vi "CR test.vi"() -> ()   [LabVIEW 2021]
uses:
  Data Model/ELAN Data Model/Type Definitions/Value full.ctl
  Data Unit/ELAN PC Data Unit/Elan units.ctl
  Data Unit/ELAN PC Data Unit/Elan measured variable.ctl
  Data Unit/ELAN PC Data Unit/Elan channel state.ctl
  enums/main_prog_state.ctl
  enums/init_state.ctl
  Master CR.lvclass
  Param/TCP Param/TCP Param.lvclass
  D:/my_projects/projects/Algorithms/Labview/21/Master CR/Param/Param.lvclass
  Master CR.lvclass/Master CR.ctl
  Param/Param.lvclass/Param.ctl
  Param/TCP Param/TCP Param.lvclass/TCP Param.ctl
  <vilib>/Platform/TimedLoop/XDataNode/timing_clust.ctl
  <vilib>/Platform/TimedLoop/XDataNode/nitl_modes.ctl
  <vilib>/Platform/TimedLoop/XDataNode/wakeup.ctl
  Data Model/ELAN Data Model/ELAN Data Model.lvclass
  enums/close_state.ctl
  <vilib>/Platform/TimedLoop/XDataNode/XDataNode.xnode
  Modbus_v121c/Data Model/Device Data Model.lvclass
  <vilib>/Platform/TimedLoop/XDataNode/XDNodeRunTimeDep.lvlib
  enums/Param_MB test.lvlib
  Param/Param.lvclass
  Data Unit/ELAN PC Data Unit/ELAN PDU.lvclass
panel:
  out "Values":T1[][](array[typedef]) {"Value"."Value" format="%#_6f"}
  in  "Write":bool
  in  "Read":bool
  out "connects":bool[](array[boolean])
  out "DI":bool[][](array[boolean])
  out "AI":u16[][](array[numeric])
  in  "DO":bool[][](array[boolean])
  in  "AOint":u16[][](array[numeric])
  out "comm error":errorcluster
  out "initialise error":errorcluster
  in  "EP_on":bool
  in  "tick":i64=100 caption="Время цикла основной программы" min=5 max=500 step=1
  in  "stop":bool
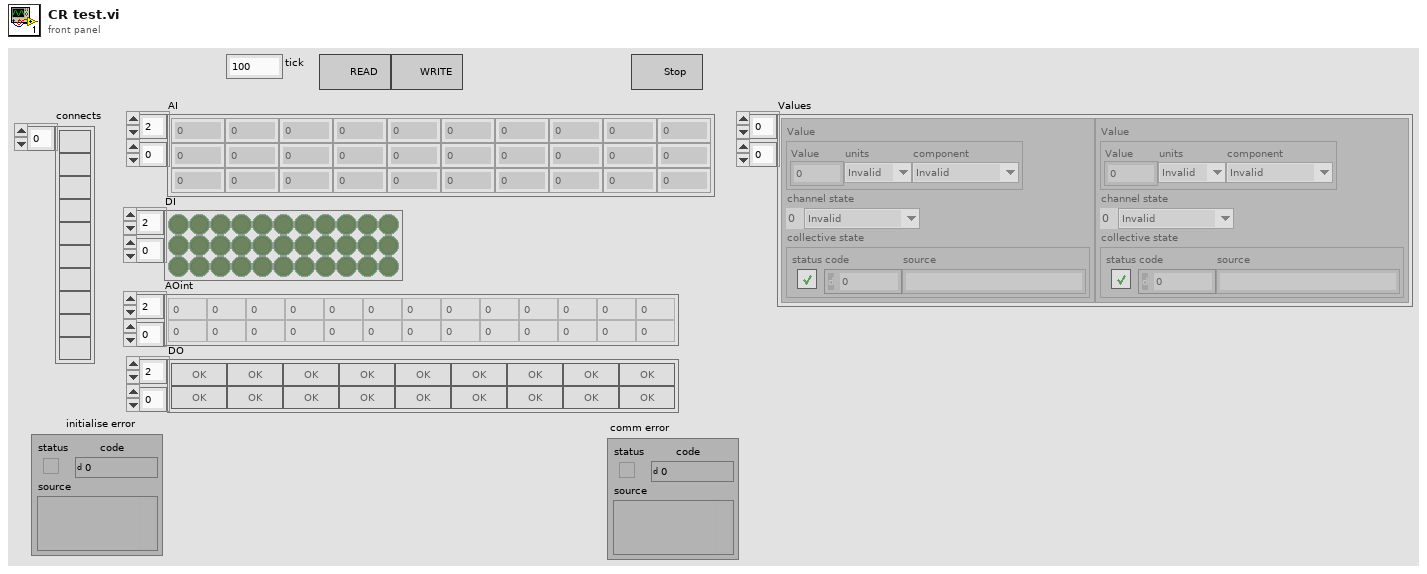
[diagram p1: front panel]
types:
  T1 = typedef "ELAN Data Model.lvclass/Value full.ctl" = cluster{"Value":cluster{"Value":sgl, "units":T2, "component":T3}, "channel state":T4, "collective state":errorcluster}
  T2 = typedef "ELAN PDU.lvclass/Elan units.ctl" = enum16{"Invalid", "no dimension", "ppm", "ppb", "vpm", "ppm C1", "ppm C3", "ppm C6", "mg C/m3", "mg/m3", "%", "% vol", "% of measuring range", "% saturation", "%/°C", "%/K", "% weight", "mV/pH", "mV/mbar", "nA/mbar", "S/m", "S/cm", "mS/m", "mS/cm", "мS/m", "мS/cm", "S", "min", "H", "Pa", "MA", "uV", "MV", "V", "mbar", "hPa", "Ml/min", "kOhm", "MOhm", "S1", "°C", "Hz", "pH", "ug/l", "mg/l", "l/min", "uA", "mg/dm3", "kPa", "kOhm*cm", "MOhm*cm", "°", "1/min", "1/m", "g/m3", "g/l", "% Vol C"}
  T3 = typedef "ELAN PDU.lvclass/Elan measured variable.ctl" = enum16{"Invalid", "no component", "CO", "CO2", "CH4 (Methan)", "C6H14 (Hexan)", "SO2", "NO", "NO2", "CHClF2 (R22)", "C3H8 (Propan)", "C4H10 (Butan)", "O2", "C5H12 (Pentan)", "CnHm (THC)", "P (process pressure)", "pH", "T (temperature)", "C2H4 (Ethen)", "C2H2 (Ethin)", "C3H6 (Propen)", "C4H6", "C4H8", "C2H6", "NH3 (Ammoniak)", "N2O", "C6H6 (Benzol)", "SF6", "CH3OH (Methanol)", "C2H5OH (Ethanol)", "CH2Cl2", "C2H4Cl2", "CH3Cl", "C2H4O", "H2O (water vapor)", "G/l (conductivity)", "C", "S", "N", "CF4", "COCl2 (phosgene)", "CHF3 (R23)", "C2F6 (R116)", "------ (self defined component)", "C2H3Cl", "H2 (Hydrogen)", "Ar", "He", "Cl2", "N2"}
  T4 = typedef "ELAN PDU.lvclass/Elan channel state.ctl" = enum16{"Invalid", "Warm-up", "Pause", "Standby", "Measure", "Zero calibration", "Adjust component slope", "Not yet defined1", "Adjust curve dip", "Adjust linearization sensitivity", "Adjust temperature compensation", "Adjust pressure compensation", "Adjust linearization zero", "Not yet defined2", "Autocal", "Adjust phase", "Zero calibration of O2 sensor", "Synchronous zero calibration", "Purging for synchronous zero calibration", "Adjust analog output", "Adjust analog input", "Autocal check"}
  T5 = cluster{"conn_timeout":i32, "reconn_timeout":i32, "N attempt max":i32, "t_reset_TTL":i32, "write_timeout":i32, "read_timeout":i32, "period":i32}[]
  T6 = cluster{"Remote IP Address":string, "Remote Port":u16}[]
  T7 = typedef "Param_MB test.lvlib/init_state.ctl" = enum16{"Init Data", "Init TMPs", "Init system DB", "Init data DB", "Read Enums", "Init arrays", "Init KFM", "Init Param", "Init AI param", "Init DI param", "Init AO param", "Init DO param", "Init ALR param", "Init save progs", "Read OPC param", "Init Shared Variables", "Init regulators", "Init heaters", "Init Y defs", "Exit"}
  T8 = typedef "Param_MB test.lvlib/main_prog_state.ctl" = enum16{"Read_AI_Param", "Read_DI_Param", "Read_AO_Param", "Read_DO_Param", "Read_ALR_ON_OFF", "Read_ALR_Param", "Read_Param", "Read_REG_Param", "Timers", "AI", "DI", "SendAItoScada", "SendDItoScada", "Alarms", "SendAItoDB", "SendDItoDB", "SendALRtoDB", "Messages", "Controls", "Control HT1", "QN_control", "QN", "QN_state", "Control EB3", "Outputs", "Exit"}
  T9 = cluster{"KFM":string[], "PAR":string[], "AI":string[], "DI":string[], "DI_fast":string[], "AO":string[], "Regs":string[], "DO":string[], "ALR":string[], "System":string[]}
  T10 = cluster{"Enums":cluster{"KFM":string[], "PAR":string[], "AI":string[], "DI":string[], "DI_fast":string[], "AO":string[], "Regs":string[], "DO":string[], "ALR":string[], "System":string[]}, "MBs":refnum<class "Master CR.lvclass">[]}
  T11 = cluster{"current time":timestamp, "Timer_1s":bool, "Timer_10s":bool, "Timer_1day":bool}
  T12 = typedef "XDNodeRunTimeDep.lvlib/timing_clust.ctl" = cluster{"Expected End [f-1]":u64, "Actual End [f-1]":u64, "Finished Late? [f-1]":bool, "Expected End [i-1]":u64, "Actual End [i-1]":u64, "Finished Late? [i-1]":bool, "Expected Start [i]":u64, "Actual Start [i]":u64, "Expected Start [f]":u64, "Actual Start [f]":u64, "Source Name":string, "Structure Name":string, "Period":i64, "Deadline":i64, "Offset":i64, "Start":i64, "Priority":i32, "Timeout":i32, "Mode":T13, "Wakeup Reason":T14, "Error":errorcluster, "Source Type":string, "Secondary Source Type":string, "Global End Time":u64, "Global Start Time":u64, "Frame Duration":u64, "Iteration Duration":u64, "Assigned CPU":i32, "I/O Scan Engine Mode":u32}
  T13 = typedef "XDNodeRunTimeDep.lvlib/nitl_modes.ctl" = enum32{"No Change", "Process missed periods, maintain original phase", "Discard missed periods, maintain original phase", "Process missed periods, ignore original phase", "Discard missed periods, ignore original phase"}
  T14 = typedef "XDNodeRunTimeDep.lvlib/wakeup.ctl" = enum32{"Normal", "Aborted", "Asynchronous wakeup", "Timing source error", "Timed loop error", "Timeout"}
  T15 = typedef "Param_MB test.lvlib/close_state.ctl" = enum16{"QN_state notifier", "QN_control_queue", "ALR notifires", "ALR", "DO notifires", "DO", "AO notifires", "AO", "DI notifres", "DI", "AI notifires", "AI", "OPC", "Param", "SaveMessageProg", "KFM DadaRef", "KFM Registers", "KFM StatusRef", "Exit"}
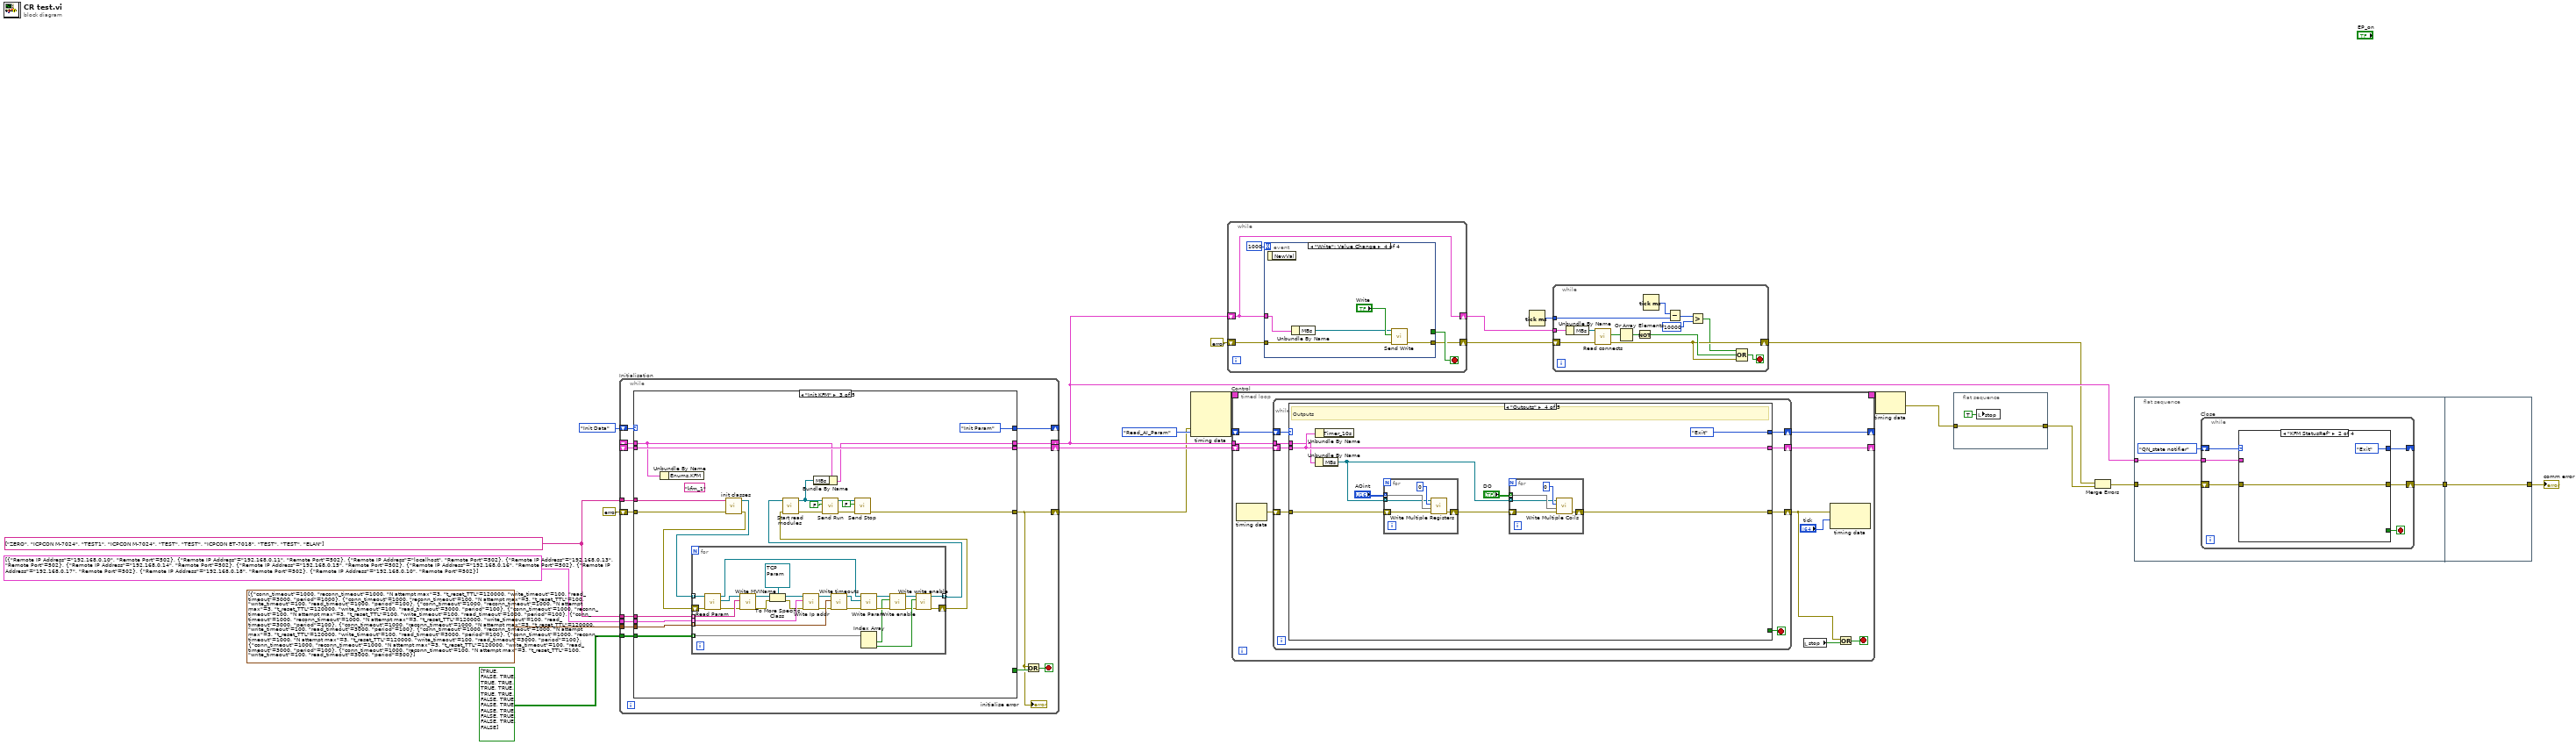
[diagram p0: block diagram]
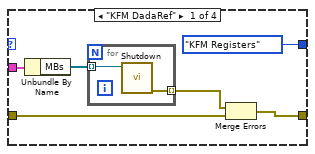
[diagram p2: hidden frame]
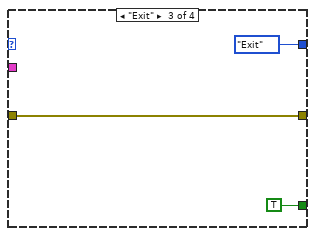
[diagram p3: hidden frame]
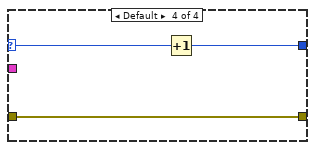
[diagram p4: hidden frame]
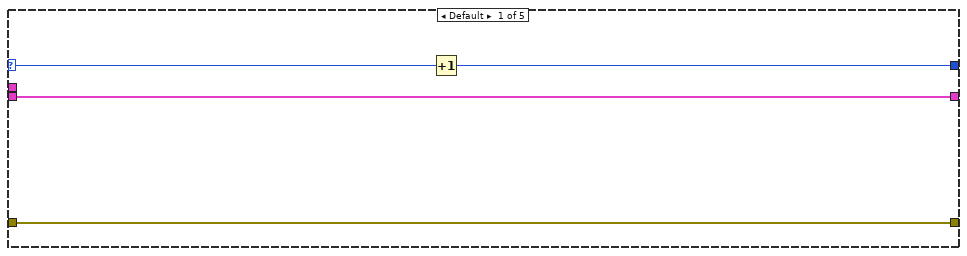
[diagram p5: hidden frame]
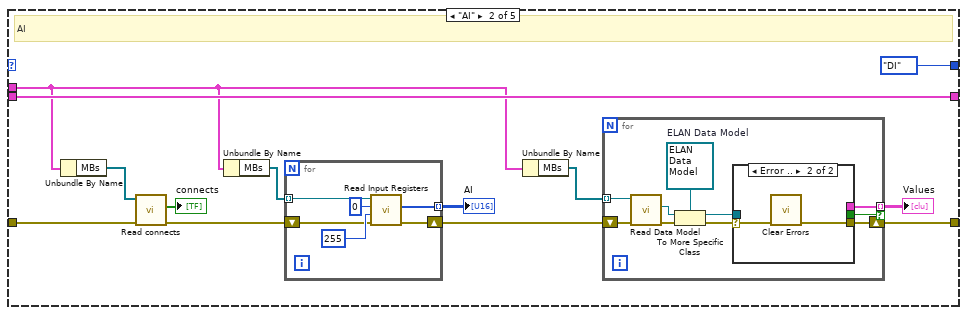
[diagram p6: hidden frame]
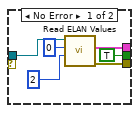
[diagram p7: hidden frame]
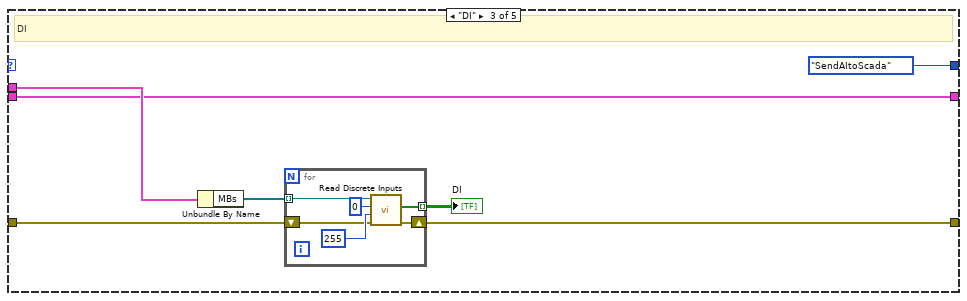
[diagram p8: hidden frame]
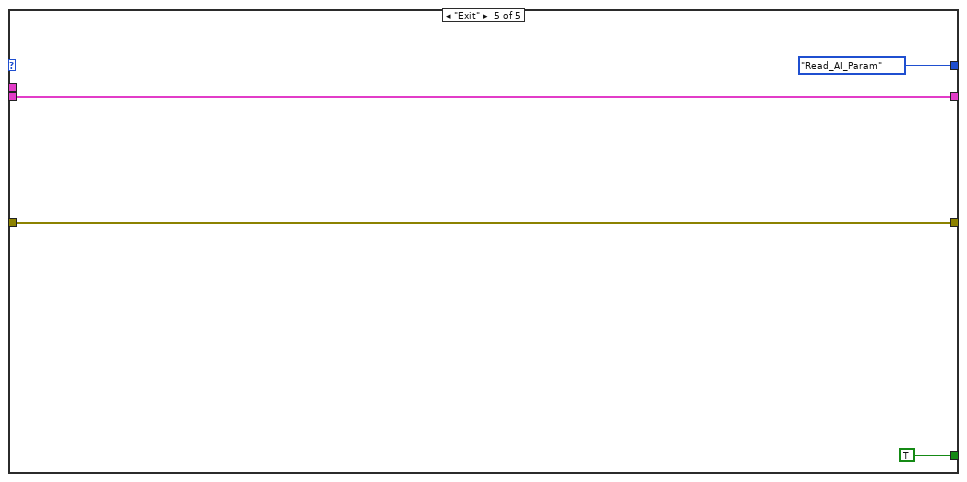
[diagram p9: hidden frame]
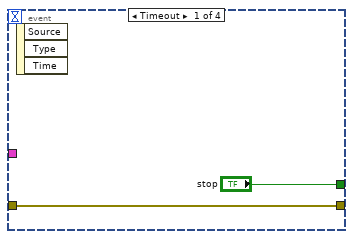
[diagram p10: hidden frame]
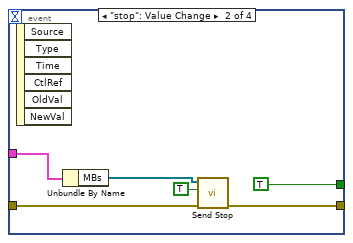
[diagram p11: hidden frame]
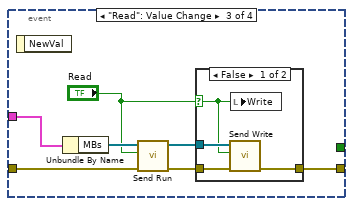
[diagram p12: hidden frame]
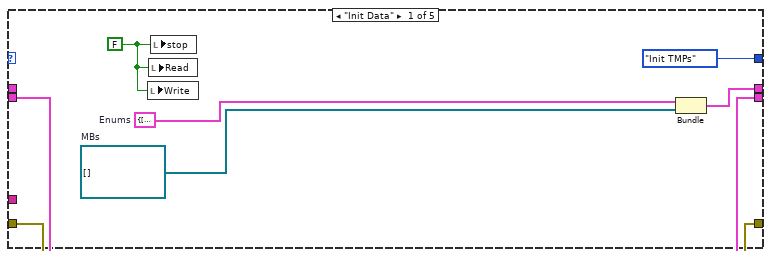
[diagram p14: hidden frame]
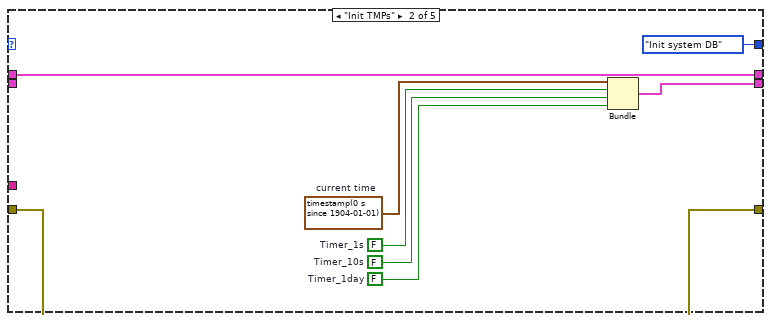
[diagram p15: hidden frame]
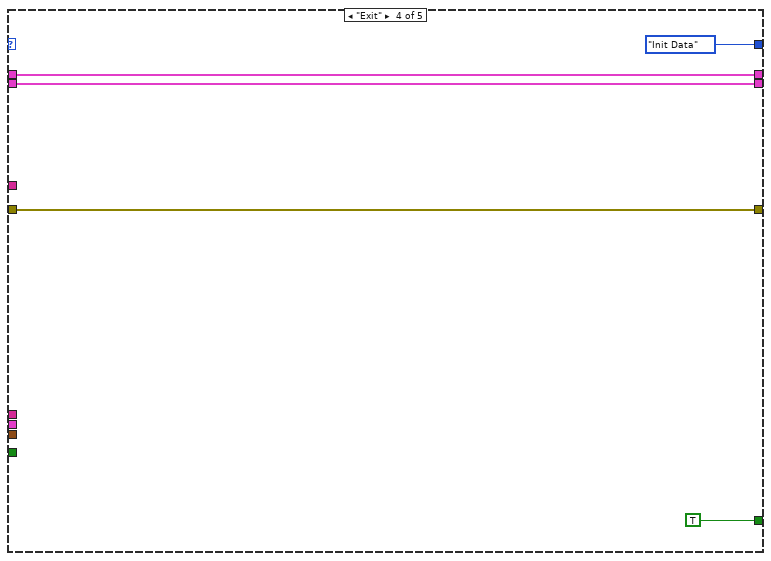
[diagram p16: hidden frame]
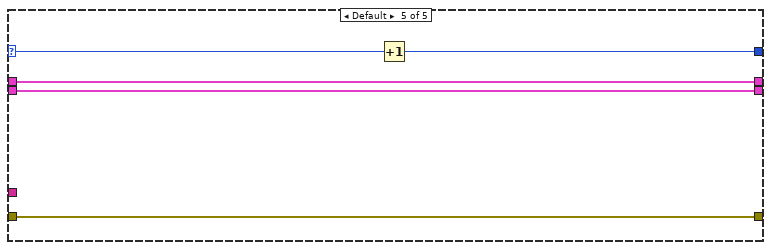
[diagram p17: hidden frame]
diagram:
  w8 = string[] ["ZERO", "ICPCON M-7024", "TEST1", "ICPCON M-7024", "TEST", "TEST", "ICPCON ET-7018", "TEST", "TEST", "ELAN"] ("MVIName")
  n1 = while "Initialisation" {
    shift-right: [w28] -> w7
    shift-left: errorcluster {"status"=FALSE, "code"=0, "source"=""} ("error out") -> [w34]
    shift-right: [w37] -> w13
    shift-left: _ -> [w35]
    shift-right: [w33] -> _
    shift-left: init_state."Init Data" -> [w36]
    shift-right: [w30] -> w16
    shift-left: _ -> [w29]
    tunnel: w8 -> [w27]
    tunnel: T6 [{"Remote IP Address"="192.168.0.10", "Remote Port"=502}, {"Remote IP Address"="192.168.0.11", "Remote Port"=502}, {"Remote IP Address"="localhost", "Remote Port"=502}, {"Remote IP Address"="192.168.0.13", "Remote Port"=502}, {"Remote IP Address"="192.168.0.14", "Remote Port"=502}, {"Remote IP Address"="192.168.0.15", "Remote Port"=502}, {"Remote IP Address"="192.168.0.16", "Remote Port"=502}, {"Remote IP Address"="192.168.0.17", "Remote Port"=502}, {"Remote IP Address"="192.168.0.18", "Remote Port"=502}, {"Remote IP Address"="192.168.0.10", "Remote Port"=502}] ("IP Address") -> [w26]
    tunnel: T5 [{"conn_timeout"=1000, "reconn_timeout"=1000, "N attempt max"=3, "t_reset_TTL"=120000, "write_timeout"=100, "read_timeout"=3000, "period"=1000}, {"conn_timeout"=1000, "reconn_timeout"=100, "N attempt max"=3, "t_reset_TTL"=100, "write_timeout"=100, "read_timeout"=1000, "period"=100}, {"conn_timeout"=1000, "reconn_timeout"=1000, "N attempt max"=3, "t_reset_TTL"=120000, "write_timeout"=100, "read_timeout"=3000, "period"=100}, {"conn_timeout"=1000, "reconn_timeout"=100, "N attempt max"=3, "t_reset_TTL"=100, "write_timeout"=100, "read_timeout"=1000, "period"=100}, {"conn_timeout"=1000, "reconn_timeout"=1000, "N attempt max"=3, "t_reset_TTL"=120000, "write_timeout"=100, "read_timeout"=3000, "period"=100}, {"conn_timeout"=1000, "reconn_timeout"=1000, "N attempt max"=3, "t_reset_TTL"=120000, "write_timeout"=100, "read_timeout"=3000, "period"=100}, {"conn_timeout"=1000, "reconn_timeout"=1000, "N attempt max"=3, "t_reset_TTL"=120000, "write_timeout"=100, "read_timeout"=3000, "period"=100}, {"conn_timeout"=1000, "reconn_timeout"=1000, "N attempt max"=3, "t_reset_TTL"=120000, "write_timeout"=100, "read_timeout"=3000, "period"=100}, {"conn_timeout"=1000, "reconn_timeout"=1000, "N attempt max"=3, "t_reset_TTL"=120000, "write_timeout"=100, "read_timeout"=3000, "period"=100}, {"conn_timeout"=1000, "reconn_timeout"=100, "N attempt max"=3, "t_reset_TTL"=100, "write_timeout"=100, "read_timeout"=3000, "period"=500}] ("timeouts") -> [w25]
    tunnel: bool[][] [[TRUE, FALSE], [TRUE, TRUE], [TRUE, TRUE], [TRUE, TRUE], [TRUE, FALSE], [TRUE, FALSE], [TRUE, FALSE], [TRUE, FALSE], [TRUE, FALSE], [TRUE, FALSE]] ("enable") -> [w24]
    tunnel: w8 -> [w23]
    stop <- w31 stop-if-true
    # "Initialisation"
    n2 = case shown="\"Init KFM\"" w36 {
      tunnel: [w42 w51 w53 w102 w105] -> w28
      selector: w36 -> [_ _ _ _ w108]
      tunnel: [w43 w50 w54 w103 w106] -> w37
      tunnel: w35 -> [_ w50 w71 w103 w106]
      tunnel: w34 -> [w42 w51 w70 w102 w105]
      tunnel: [init_state."Init TMPs" init_state."Init system DB" init_state."Init Param" init_state."Init Data" w107] -> w33
      tunnel: [_ _ _ TRUE _] -> w32
      tunnel: [w40 w49 w72 w100 w109] -> w30
      tunnel: w29 -> [w40 _ w72 w100 w109]
      tunnel: w27 -> [_ _ w65 _ _]
      tunnel: w26 -> [_ _ w64 _ _]
      tunnel: w25 -> [_ _ w63 _ _]
      tunnel: w24 -> [_ _ w62 _ _]
      tunnel: w23 -> [_ _ w61 _ _]
      frame "Init Data" {
        w38 = FALSE ("stop")
        w39 = refnum<class "Master CR.lvclass">[] []  # MBs
        w41 = T9 {"KFM"=[], "PAR"=[], "AI"=[], "DI"=[], "DI_fast"=[], "AO"=[], "Regs"=[], "DO"=[], "ALR"=[], "System"=[]}  # Enums
        n3 = local write "Write"(w38) -> ()
        n4 = local write "Read"(w38) -> ()
        n5 = local write "stop"(w38) -> ()
        n6 = Bundle("Enums"=w41, "MBs"=w39) -> (w43:T10)  [unwired: 1 in]
      }
      frame "Init TMPs" {
        w45 = FALSE  # Timer_10s
        w46 = FALSE  # Timer_1day
        w47 = FALSE  # Timer_1s
        w48 = timestamp(0 s since 1904-01-01)  # current time
        n7 = Bundle("current time"=w48, "Timer_1s"=w47, "Timer_10s"=w45, "Timer_1day"=w46) -> (w49:T11)  [unwired: 1 in]
      }
      frame "Init KFM" {
        (unwired) "kfm_1" ("KFMTable")
        n8 = Unbundle By Name(w71) -> ()  [unwired: 1 out]
        n9 = call "init classes.vi"("error in (no error)"=w70, "MVINames"=w61) -> ("error out"=w67:errorcluster, "MBs"=w69:refnum<class "Master CR.lvclass">[])  [unwired: 8 in]
        n10 = for {
          tunnel: w69 -> [w75] mode=indexing
          tunnel: w64 -> [w82] mode=indexing
          tunnel: w63 -> [w79] mode=indexing
          tunnel: w65 -> [w97] mode=indexing
          tunnel: w62 -> [w91] mode=indexing
          tunnel: [w87] -> w68 mode=indexing
          shift-right: [w86] -> w66
          shift-left: w67 -> [w99]
          n11 = call "Read Param.vi"("error in (no error)"=w99, "MB_TCP in"=w75) -> ("error out"=w95:errorcluster, "Param"=w74:refnum<class "Param.lvclass">, "MB_TCP out"=w94:refnum<class "Master CR.lvclass">)  [unwired: 7 in]
          n12 = call "Write MVIName.vi"("error in (no error)"=w95, "MVIName"=w97, "MB Param in"=w74) -> ("error out"=w84:errorcluster, "MB Param out"=w96:refnum<class "Param.lvclass">)  [unwired: 7 in]
          n13 = To More Specific Class(target class=refnum<class "TCP Param.lvclass"> refnum ("Param.lvlib:TCP Param.lvclass"), reference=w96, error in=w84) -> (specific class reference=w83:refnum<class "TCP Param.lvclass">, error out=w81:errorcluster)
          n14 = call "Write Ip addr.vi"("error in (no error)"=w81, "IP address"=w82, "MB Param in"=w83) -> ("error out"=w78:errorcluster, "MB Param out"=w80:refnum<class "TCP Param.lvclass">)  [unwired: 7 in]
          n15 = call "Write timeouts.vi"("error in (no error)"=w78, "timeouts"=w79, "MB Param in"=w80) -> ("error out"=w77:errorcluster, "MB Param out"=w76:refnum<class "TCP Param.lvclass">)  [unwired: 7 in]
          n16 = call "Write Param.vi"("error in (no error)"=w77, "Param"=w76, "MB_TCP in"=w94) -> ("error out"=w92:errorcluster, "MB_TCP out"=w93:refnum<class "Master CR.lvclass">)  [unwired: 7 in]
          n17 = Index Array(array=w91) -> (element #1=w90:bool, element #2=w89:bool)  [unwired: 2 in]
          n18 = call "Write enable.vi"("error in (no error)"=w92, "enable"=w90, "Master CR in"=w93) -> ("error out"=w88:errorcluster, "Master CR out"=w98:refnum<class "Master CR.lvclass">)  [unwired: 7 in]
          n19 = call "Write write enable.vi"("error in (no error)"=w88, "write enable"=w89, "Master CR in"=w98) -> ("error out"=w86:errorcluster, "Master CR out"=w87:refnum<class "Master CR.lvclass">)  [unwired: 7 in]
        }
        n20 = call "Start read modules.vi"("error in"=w66, "classes"=w68) -> ("error out"=w56:errorcluster, "classes initialised"=w55:refnum<class "Master CR.lvclass">[])  [unwired: 8 in]
        n21 = Bundle By Name(cluster=w71, "MBs"=w55) -> (w54:T10)
        n22 = call "Send Run.vi"("error in"=w56, "Run"=FALSE, "MCRs"=w55) -> ("error out"=w59:errorcluster, "MCRs out"=w60:refnum<class "Master CR.lvclass">[])  [unwired: 7 in]
        n23 = call "Send Stop.vi"("error in"=w59, "Stop"=FALSE ("Write"), "MCRs"=w60) -> ("error out"=w53:errorcluster)  [unwired: 7 in, 1 out]
      }
      frame "Exit" {
      }
      frame Default {
        n24 = Increment(x=w108) -> (x+1=w107:T7)
      }
    }
    "initialise error" <- w28
    n25 = Or(x=w28, y=w32) -> (x .or. y?=w31:bool)
  }
  n26 = node-c288(w7) -> (w22:T12)  [unwired: 3 in]
  n27 = while {
    shift-right: [w112] -> w4
    shift-left: errorcluster {"status"=FALSE, "code"=0, "source"=""} ("error out") -> [w111]
    shift-right: [w110] -> w3
    shift-left: w13 -> [w110]
    stop <- w113 stop-if-true
    n28 = event shown="[3] \"Write\": Value Change" {
      selector: _ -> [_ _ _ _]
      dyn-events: _ -> [_ _ _ _]
      timeout: 1000 -> [_ _ _ _]
      tunnel: ["stop" TRUE ("stop") _ _] -> w113
      tunnel: w110 -> [_ w117 w129 w139]
      tunnel: w111 -> [w115 w121 w128 w138]
      tunnel: [w115 w120 w123 w137] -> w112
      event Timeout {
        n29 = event-data() -> ()  [unwired: 1 in, 3 out]
      }
      event "stop": Value Change {
        n30 = event-data() -> ()  [unwired: 1 in, 6 out]
        n31 = Unbundle By Name(w117) -> ("MBs"=w118:refnum<class "Master CR.lvclass">[])
        n32 = call "Send Stop.vi"("error in"=w121, "Stop"=TRUE, "MCRs"=w118) -> ("error out"=w120:errorcluster)  [unwired: 7 in, 1 out]
      }
      event "Read": Value Change {
        n33 = event-data() -> ()  [unwired: 1 in, 1 out]
        n34 = Unbundle By Name(w129) -> ("MBs"=w127:refnum<class "Master CR.lvclass">[])
        n35 = call "Send Run.vi"("error in"=w128, "Run"="Read", "MCRs"=w127) -> ("error out"=w125:errorcluster, "MCRs out"=w124:refnum<class "Master CR.lvclass">[])  [unwired: 7 in]
        n36 = case shown="False" "Read" {
          selector: "Read" -> [w131 _]
          tunnel: w125 -> [w133 w134]
          tunnel: w124 -> [w132 _]
          tunnel: [w130 w134] -> w123
          frame False {
            n37 = call "Send Write.vi"("error in"=w133, "Write"=w131, "MCRs"=w132) -> ("error out"=w130:errorcluster)  [unwired: 7 in, 1 out]
            n38 = local write "Write"(w131) -> ()
          }
          frame True {
          }
        }
      }
      event "Write": Value Change {
        n39 = event-data() -> ()  [unwired: 1 in, 1 out]
        n40 = Unbundle By Name(w139) -> ("MBs"=w135:refnum<class "Master CR.lvclass">[])
        n41 = call "Send Write.vi"("error in"=w138, "Write"="Write", "MCRs"=w135) -> ("error out"=w137:errorcluster)  [unwired: 7 in, 1 out]
      }
    }
  }
  n42 = timed-loop "Control" {
    tunnel: w13 -> [w149]
    shift-right: [w147] -> _
    shift-left: w16 -> [w148]
    timing: w22 -> [_]
    timing-out: [_] -> w21
    shift-right: [w145] -> _
    shift-left: main_prog_state."Read_AI_Param" -> [w144]
    stop <- w142 stop-if-true
    n43 = node-c288() -> (w146:errorcluster)  [unwired: 1 in]
    n44 = while {
      tunnel: w149 -> [w157]
      shift-right: [w155] -> w147
      shift-left: w148 -> [w156]
      shift-right: [w150] -> w140
      shift-left: w146 -> [w154]
      shift-right: [w153] -> w145
      shift-left: w144 -> [w152]
      stop <- w151 stop-if-true
      n45 = case shown="\"Outputs\"" w152 {
        tunnel: w154 -> [w158 w173 w201 w217 w231]
        tunnel: w157 -> [_ w163 w204 w218 _]
        tunnel: w156 -> [w160 w171 w203 w219 w232]
        tunnel: [w160 w171 w203 w219 w232] -> w155
        selector: w152 -> [w161 _ _ _ _]
        tunnel: [w159 main_prog_state."DI" main_prog_state."SendAItoScada" main_prog_state."Exit" main_prog_state."Read_AI_Param"] -> w153
        tunnel: [_ _ _ _ TRUE] -> w151
        tunnel: [w158 w169 w200 w213 w231] -> w150
        frame Default {
          n46 = Increment(x=w161) -> (x+1=w159:T8)
        }
        frame "AI" {
          # "AI"
          n47 = Unbundle By Name(w163) -> ("MBs"=w172:refnum<class "Master CR.lvclass">[])
          n48 = call "Read connects.vi"("error in (no error)"=w173, "MCRs in"=w172) -> ("error out"=w166:errorcluster, "connects"=→"connects":bool[])  [unwired: 7 in, 1 out]
          n49 = Unbundle By Name(w163) -> ("MBs"=w164:refnum<class "Master CR.lvclass">[])
          n50 = for {
            tunnel: w164 -> [w176] mode=indexing
            shift-right: [w180] -> w165
            shift-left: w166 -> [w175]
            tunnel: [w177] -> w162 mode=indexing
            n51 = call "Read Input Registers.vi"("error in"=w175, "number of inputs"=u16 255 ("number of coils"), "starting address"=u16 0, "Master CR in"=w176) -> ("error out"=w180:errorcluster, "register values"=w177:u16[])  [unwired: 5 in, 1 out]
          }
          "AI" <- w162
          n52 = Unbundle By Name(w163) -> ("MBs"=w170:refnum<class "Master CR.lvclass">[])
          n53 = for {
            tunnel: w170 -> [w187] mode=indexing
            shift-right: [w190] -> w169
            shift-left: w165 -> [w188]
            tunnel: [w189] -> w167 mode=indexing if=w181
            w185 = refnum<class "ELAN Data Model.lvclass"> refnum  # ELAN Data Model
            n54 = call "Read Data Model.vi"("error in (no error)"=w188, "Master CR in"=w187) -> ("error out"=w186:errorcluster, "Data Model"=w184:refnum<class "Device Data Model.lvclass">)  [unwired: 7 in, 1 out]
            n55 = To More Specific Class(target class=w185, reference=w184, error in=w186) -> (specific class reference=w183:refnum<class "ELAN Data Model.lvclass">, error out=w182:errorcluster)
            n56 = case shown="Error .." w182 {
              selector: w182 -> [_ w198]
              tunnel: [w196 w197] -> w190
              tunnel: [w193 _] -> w189
              tunnel: w183 -> [w192 _]
              tunnel: [TRUE _] -> w181
              frame No Error {
                n57 = call-dynamic "Read ELAN Values.vi"("number of registers"=u16 2 ("number of coils"), "starting address"=u16 0, "standard data model in"=w192) -> ("error out"=w196:errorcluster, "Values"=w193:T1[])  [unwired: 6 in, 1 out]
              }
              frame Error {
                n58 = call <vilib>:"Clear Errors.vi"("error in (no error)"=w198) -> ("error out"=w197:errorcluster)  [unwired: 5 in, 1 out]
              }
            }
          }
          "Values" <- w167
        }
        frame "DI" {
          # "DI"
          n59 = Unbundle By Name(w204) -> ("MBs"=w202:refnum<class "Master CR.lvclass">[])
          n60 = for {
            tunnel: w202 -> [w207] mode=indexing
            shift-right: [w211] -> w200
            shift-left: w201 -> [w206]
            tunnel: [w208] -> w199 mode=indexing
            n61 = call "Read Discrete Inputs.vi"("error in"=w206, "number of inputs"=u16 255 ("number of coils"), "starting address"=u16 0, "Master CR in"=w207) -> ("error out"=w211:errorcluster, "discrete inputs"=w208:bool[])  [unwired: 5 in, 1 out]
          }
          "DI" <- w199
        }
        frame "Outputs" {
          # "Outputs"
          n62 = Unbundle By Name(w218) -> ("MBs"=w212:refnum<class "Master CR.lvclass">[])
          n63 = Unbundle By Name(w219) -> ()  [unwired: 1 out]
          n64 = for {
            tunnel: w212 -> [w226] mode=indexing
            shift-right: [w230] -> w214
            shift-left: w217 -> [w227]
            tunnel: "AOint" -> [w228] mode=indexing
            n65 = call-dynamic "Write Multiple Registers.vi"("error in"=w227, "register values"=w228, "starting address"=u16 0, "Master CR in"=w226) -> ("error out"=w230:errorcluster)  [unwired: 6 in, 1 out]
          }
          n66 = for {
            tunnel: w212 -> [w222] mode=indexing
            shift-right: [w225] -> w213
            shift-left: w214 -> [w221]
            tunnel: "DO" -> [w223] mode=indexing
            n67 = call-dynamic "Write Multiple Coils.vi"("error in"=w221, "coils"=w223, "starting address"=u16 0, "Master CR in"=w222) -> ("error out"=w225:errorcluster)  [unwired: 6 in, 1 out]
          }
        }
        frame "Exit" {
        }
      }
    }
    n68 = local read "stop"() -> (w141:bool)
    n69 = node-c288(w140, "tick") -> ()  [unwired: 1 out]
    n70 = Or(x=w140, y=w141) -> (x .or. y?=w142:bool)
  }
  n71 = Tick Count (ms)() -> (millisecond timer value=w2:u32)
  n72 = while {
    shift-right: [w246] -> w1
    shift-left: w4 -> [w253]
    tunnel: w3 -> [w250]
    tunnel: w2 -> [w244]
    stop <- w248 stop-if-true
    n73 = Unbundle By Name(w250) -> ("MBs"=w249:refnum<class "Master CR.lvclass">[])
    n74 = call "Read connects.vi"("error in (no error)"=w253, "MCRs in"=w249) -> ("error out"=w246:errorcluster, "connects"=w252:bool[])  [unwired: 7 in, 1 out]
    n75 = Or Array Elements(Boolean array=w252) -> (logical OR=w251:bool)
    n76 = Not(x=w251) -> (.not. x?=w247:bool)
    n77 = Tick Count (ms)() -> (millisecond timer value=w245:u32)
    n78 = Subtract(x=w245, y=w244) -> (x-y=w243:u32)
    n79 = Greater?(x=w243, y=u32 10000) -> (0:w241:bool)
    n80 = Compound Arithmetic op=OR(w241, w247, w246) -> (w248:bool)
  }
  n81 = node-c288(w21) -> (w6:errorcluster)
  n82 = flat-sequence {
    tunnel: [w254] -> w5
    tunnel: w6 -> [w254]
    frame #0 {
      n83 = local write "stop"(TRUE ("stop")) -> ()
    }
  }
  n84 = Merge Errors(w1, w5) -> (w15:errorcluster)
  n85 = flat-sequence {
    tunnel: w13 -> [w258]
    tunnel: w15 -> [w257]
    tunnel: [w256] -> w14
    tunnel: [w282] -> w19
    tunnel: w14 -> [w282]
    frame #0 {
      n86 = while "Close" {
        shift-right: [w264] -> _
        shift-left: close_state."QN_state notifier" ("Init_state") -> [w265]
        tunnel: w258 -> [w262]
        shift-right: [w260] -> w256
        shift-left: w257 -> [w261]
        stop <- w263 stop-if-true
        n87 = case shown="\"KFM StatusRef\"" w265 {
          selector: w265 -> [_ _ _ w281]
          tunnel: [close_state."KFM Registers" close_state."Exit" close_state."Exit" w280] -> w264
          tunnel: [_ _ TRUE _] -> w263
          tunnel: w262 -> [w271 _ _ _]
          tunnel: w261 -> [w269 w274 w277 w279]
          tunnel: [w268 w274 w277 w279] -> w260
          frame "KFM DadaRef" {
            n88 = Unbundle By Name(w271) -> ("MBs"=w267:refnum<class "Master CR.lvclass">[])
            n89 = for {
              tunnel: w267 -> [w273] mode=indexing
              tunnel: [w272] -> w266 mode=indexing
              n90 = call-dynamic "Shutdown.vi"("MB in"=w273) -> ("error out"=w272:errorcluster)  [unwired: 10 in]
            }
            n91 = Merge Errors(w266, w269) -> (w268:errorcluster)
          }
          frame "KFM StatusRef" {
          }
          frame "Exit" {
          }
          frame Default {
            n92 = Increment(x=w281) -> (x+1=w280:T15)
          }
        }
      }
    }
    frame #1 {
    }
  }
  "comm error" <- w19
